vi "Motors.vi"() -> ()   [LabVIEW 2018]
doc: "The myRIO Project template acquires acceleration data from the onboard accelerometer and displays the changes of acceleration values in a waveform chart."
uses:
  <vilib>/Studica/Studica Toolkit/Background/Mxp Selection.ctl
  <vilib>/robotics/Steering/Wheel/Rotation Direction.ctl
  <vilib>/robotics/Steering/Wheel/Wheel Parameters.ctl
  <vilib>/robotics/Steering/Omnidirectional Wheel/NI_Robotics_Omnidirectional Wheel.lvclass
  C:/Program Files (x86)/National Instruments/LabVIEW 2018/vi.lib/robotics/Steering/Wheel/NI_Robotics_Wheel.lvclass
  <vilib>/robotics/Steering/Omnidirectional Wheel/Create Omnidirectional Wheel.vi
  <vilib>/robotics/Steering/Steering Frame/Create User Defined Steering Frame.vi
  <vilib>/addons/control/pid/pid.llb/PID (DBL).vi
  <vilib>/robotics/Steering/Steering Frame/NI_Robotics_Steering Frame.lvclass
  <vilib>/robotics/Steering/Wheel/NI_Robotics_Wheel.lvclass
  <vilib>/addons/control/pid/NI_PID_pid.lvlib
panel:
  out "Etu":cluster{"initial PV":dbl, "SP:":dbl}(graph)={"initial PV"=0.0, "SP:"=-0.0}
  in  "PID gains":T1={"proportional gain (Kc)"=1.0, "integral time (Ti, min)"=0.01, "derivative time (Td, min)"=0.0} {"derivative time (Td, min)" format="%.3f"; "integral time (Ti, min)" format="%.3f"; "proportional gain (Kc)" format="%.3f"}
  in  "Reset Encoders":bool
  out "Radians/s":dbl[](array[numeric])
  out "Up":bool
  out "Down":bool
  out "Speed":dbl
  out "Q":bool
  out "E":bool
  out "D":bool
  out "S":bool
  out "A":bool
  out "W":bool
  out "Keys":i16[](array[numeric])
  in  "Control Type":string(combo)="Keyboard"
  in  "Stop Button":bool
  in  "Angular Velocity (rad/s)":dbl(slide) min=-1.0 max=1.0 scale=1.0..-1.0
  out "Angular Velocity Feedback":dbl(slide) scale=1.0..-1.0
  in  "Y Velocity (m/s)":dbl(slide) min=-1.0 max=1.0 scale=-1.0..1.0
  out "Y Velocity Feedback":dbl(slide) scale=-1.0..1.0
  in  "X Velocity (m/s)":dbl(slide) min=-1.0 max=1.0 scale=-1.0..1.0
  out "X Velocity Feedback":dbl(slide) scale=-1.0..1.0
  in  "Not-Connected":dbl(slide) scale=-1.0..1.0
  in  "Oikea":dbl(slide)=-0.0 scale=-1.0..1.0
  in  "Vasen":dbl(slide)=-0.0 scale=-1.0..1.0
  in  "Etu":dbl(slide)=-0.0 scale=-1.0..1.0
  # "Keyboard"
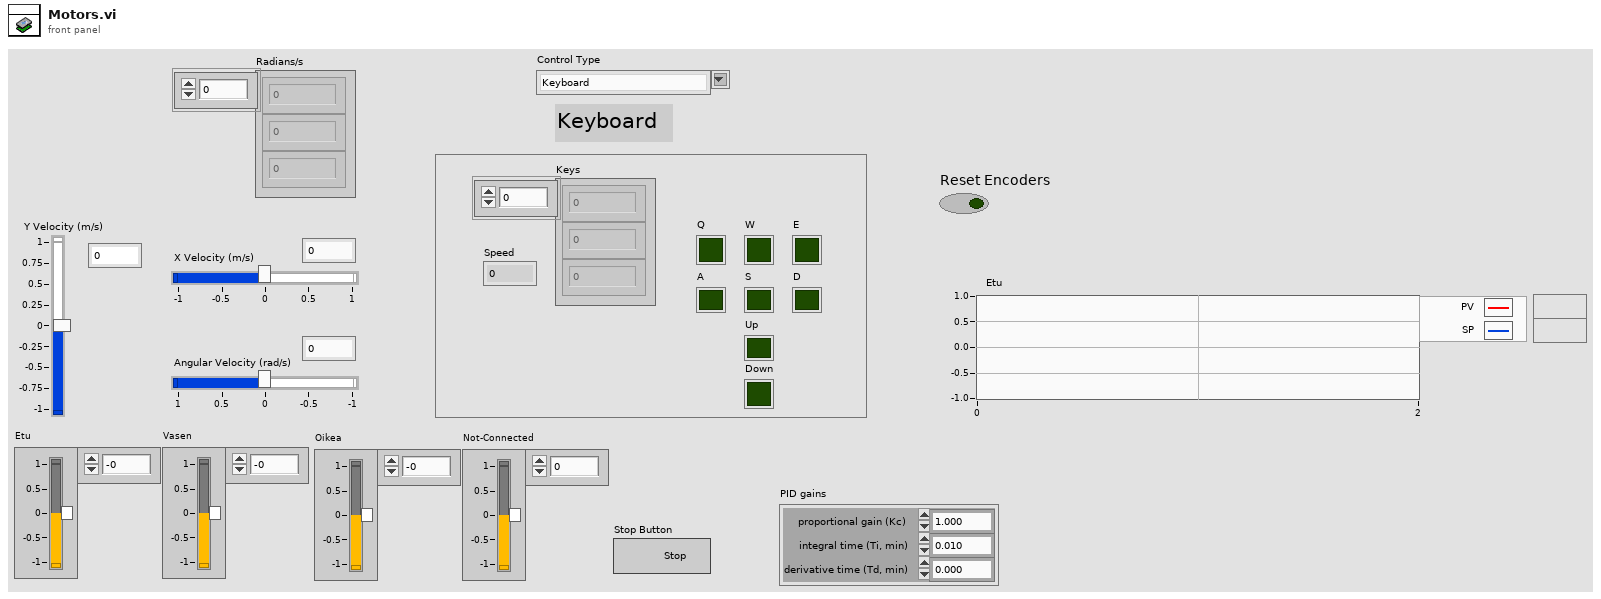
[diagram p1: front panel]
types:
  T1 = cluster{"proportional gain (Kc)":dbl, "integral time (Ti, min)":dbl, "derivative time (Td, min)":dbl}
  T2 = typedef "Mxp Selection.ctl" = enum16{"MXP A", "MXP B"}
  T3 = cluster{bool, "Tick Count(uSec)":u32, "Counter Value":i32[], "x-y":i32[]}
  T4 = typedef "NI_Robotics_Wheel.lvclass/Wheel Parameters.ctl" = cluster{"wheel radius":dbl, "gear ratio":dbl, "forward rotation direction":T5}
  T5 = typedef "NI_Robotics_Wheel.lvclass/Rotation Direction.ctl" = u16
  T6 = cluster{"Position":i32[], "Velocity RPM":dbl[], "Velocity RPS":dbl[], "Radians/s":dbl[]}
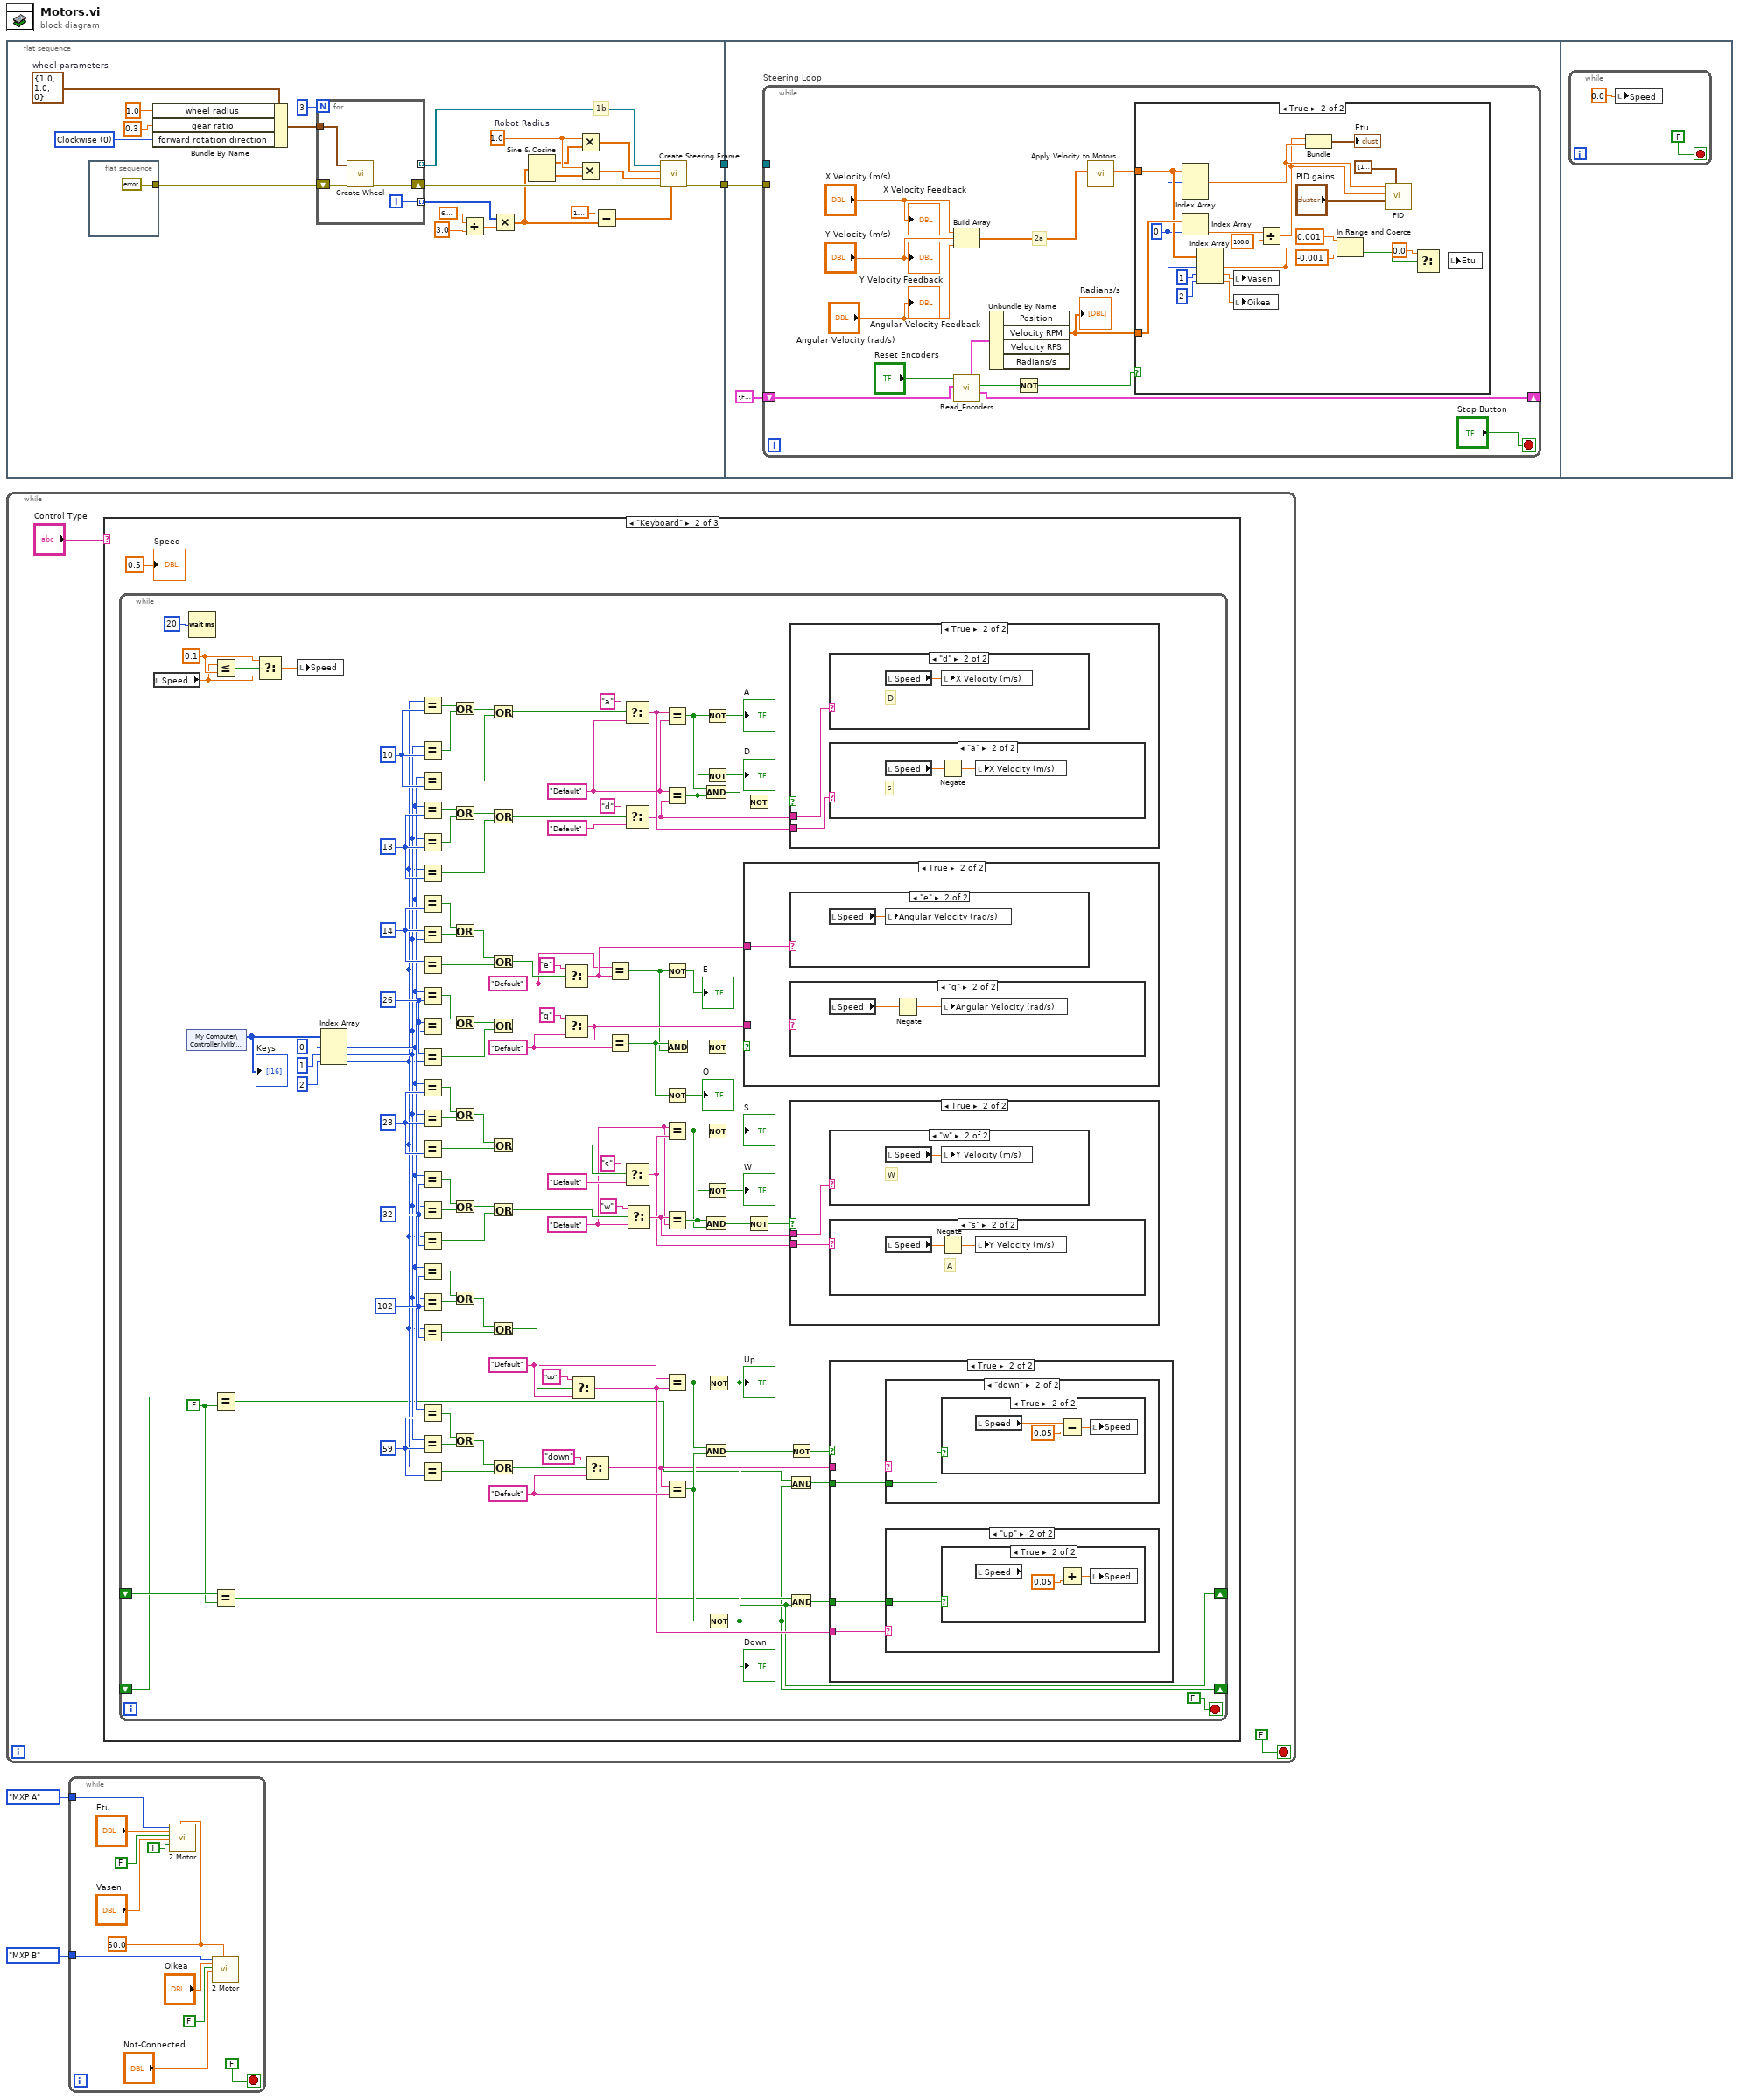
[diagram p0: block diagram]
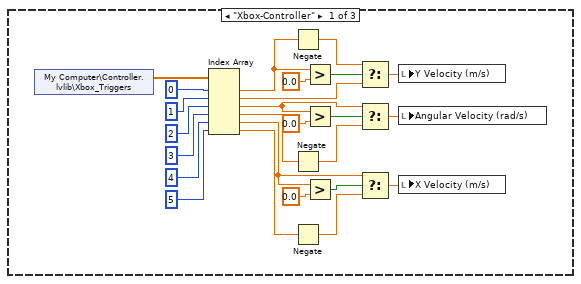
[diagram p3: hidden frame]
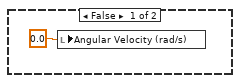
[diagram p9: hidden frame]
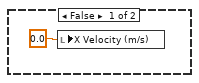
[diagram p12: hidden frame]
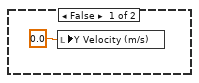
[diagram p15: hidden frame]
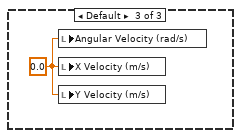
[diagram p18: hidden frame]
diagram:
  n1 = flat-sequence {
    tunnel: [w27] -> w2
    tunnel: [w8] -> w1
    tunnel: w2 -> [w34]
    tunnel: w1 -> [w36]
    frame #0 {
      w26 = T4 {"wheel radius"=1.0, "gear ratio"=1.0, "forward rotation direction"=0}  # wheel parameters
      w11 = T5 0 items=["Clockwise", "Counterclockwise"] ("forward rotation direction")
      w16 = 1.0  # Robot Radius
      # "1b"
      n2 = flat-sequence {
        tunnel: [errorcluster {"status"=FALSE, "code"=0, "source"=""} ("error out")] -> w22
        frame #0 {
        }
      }
      n3 = Bundle By Name(cluster=w26, "wheel radius"=1.0, "gear ratio"=0.3, "forward rotation direction"=w11) -> (w23:T4)
      n4 = for {
        N: 3 -> [_]
        shift-right: [w32] -> w9
        shift-left: w22 -> [w33]
        tunnel: [w31] -> w21 mode=indexing
        tunnel: w23 -> [w30]
        tunnel: [w29] -> w17 mode=indexing
        i -> [w29]
        n5 = call-poly <vilib>:"Create Wheel.vi"("error in (no error)"=w33, "wheel parameters"=w30) -> ("error out"=w32:errorcluster, "omni wheel out"=w31:refnum<class "NI_Robotics_Omnidirectional Wheel.lvclass">)  [unwired: 8 in]
      }
      n6 = Divide(x=6.283185307179586, y=3.0) -> (x/y=w18:dbl)
      n7 = Multiply(x=w17, y=w18) -> (x*y=w7:dbl[])
      n8 = Sine & Cosine(0:w7) -> (1:w6:dbl[], 2:w5:dbl[])
      n9 = Multiply(x=w16, y=w6) -> (x*y=w15:dbl[])
      n10 = Multiply(x=w16, y=w5) -> (x*y=w14:dbl[])
      n11 = Subtract(x=1.5707963267948966, y=w7) -> (x-y=w12:dbl[])
      n12 = call-poly <vilib>:"Create Steering Frame.vi"("wheel frame angles (rad)"=w12, "error in (no error)"=w9, "wheel y positions"=w14, "wheel x positions"=w15, "wheels"=w21) -> ("error out"=w8:errorcluster, "steering frame out"=w27:refnum<class "NI_Robotics_Steering Frame.lvclass">)  [unwired: 5 in]
    }
    frame #1 {
      n13 = while "Steering Loop" {
        tunnel: w36 -> [_]
        shift-right: [w42] -> _
        shift-left: T3 {FALSE, "Tick Count(uSec)"=0, "Counter Value"=[0, 0, 0, 0], "x-y"=[0, 0, 0, 0]} ("Cluster in") -> [w44]
        tunnel: w34 -> [w45]
        stop <- "Stop Button" stop-if-true
        # "2a"
        n14 = Build Array("X Velocity (m/s)", "Y Velocity (m/s)", "Angular Velocity (rad/s)") -> (w46:dbl[])
        n15 = call "Read_Encoders.vi"("Cluster in"=w44, "Reset Encoders"="Reset Encoders") -> ("Cluster Out"=w42:T3, "Updated"=w41:bool, "output cluster"=w43:T6)  [unwired: 5 in, 2 out]
        n16 = Unbundle By Name(w43) -> ("Velocity RPM"=w38:dbl[])  [unwired: 3 out]
        "Radians/s" <- w38
        n17 = Not(x=w41) -> (.not. x?=w40:bool)
        n18 = call-poly <vilib>:"Apply Velocity to Motors.vi"("steering frame velocity"=w46, "steering frame in"=w45) -> ("ccw motor velocity setpoints"=w39:dbl[])  [unwired: 5 in, 4 out]
        n19 = case shown="True" w40 {
          tunnel: w38 -> [_ w70]
          tunnel: w39 -> [_ w62]
          frame False {
          }
          frame True {
            w61 = 0 ("index")
            n20 = Index Array(array=w62, index #1=w61) -> (element #1=w67:dbl)  [unwired: 2 in, 2 out]
            n21 = Index Array(array=w70, index=w61) -> (element=w65:dbl)
            n22 = Index Array(array=w62, index #1=w61, index #2=1 ("index"), index #3=2 ("index")) -> (element #1=w51:dbl, element #2=w58:dbl, element #3=w57:dbl)
            n23 = local write "Vasen"(w58) -> ()
            n24 = local write "Oikea"(w57) -> ()
            n25 = Divide(x=w65, y=100.0) -> (x/y=w63:dbl)
            n26 = Bundle(w63, "Numeric"=w67) -> (→"Etu":cluster{dbl, "Numeric":dbl})  [unwired: 1 in]
            n27 = In Range and Coerce(upper limit=0.001, x=w51, lower limit=-0.001 ("upper limit")) -> (In Range?=w54:bool)  [unwired: 1 out]
            n28 = call-poly <vilib>:"PID.vi"("output range"=cluster{"output high":dbl, "output low":dbl} {"output high"=1.0, "output low"=-1.0}, "PID gains"="PID gains", "process variable"=w63, "setpoint"=w67) -> ()  [unwired: 6 in, 2 out]
            n29 = Select(t=0.0, s=w54, f=w51) -> (s? t:f=w52:dbl)
            n30 = local write "Etu"(w52) -> ()
          }
        }
        "X Velocity Feedback" <- "X Velocity (m/s)"
        "Y Velocity Feedback" <- "Y Velocity (m/s)"
        "Angular Velocity Feedback" <- "Angular Velocity (rad/s)"
      }
    }
    frame #2 {
      n31 = while {
        stop <- FALSE stop-if-true
        n32 = local write "Speed"(0.0 ("Speed")) -> ()
      }
    }
  }
  n33 = while {
    stop <- FALSE stop-if-true
    n34 = case shown="\"Keyboard\"" "Control Type" {
      frame "Xbox-Controller" {
        n35 = shared-variable "My Computer\\Controller.lvlib\\Xbox_Triggers"() -> (w99:dbl[])  [unwired: 1 in, 1 out]
        n36 = Index Array(array=w99, index #1=0 ("index"), index #2=1 ("index"), index #3=2 ("index"), index #4=3 ("index"), index #5=4 ("index"), index #6=5 ("index")) -> (element #1=w92:dbl, element #2=w91:dbl, element #3=w83:dbl, element #4=w81:dbl, element #5=w75:dbl, element #6=w76:dbl)
        n37 = Negate(x=w92) -> (-x=w93:dbl)
        n38 = Negate(x=w81) -> (-x=w82:dbl)
        n39 = Negate(x=w76) -> (-x=w77:dbl)
        n40 = Greater?(x=w92, y=0.0) -> (0:w95:bool)
        n41 = Greater?(x=w83, y=0.0) -> (0:w86:bool)
        n42 = Greater?(x=w75, y=0.0) -> (0:w80:bool)
        n43 = Select(t=w93, s=w95, f=w91) -> (s? t:f=w96:dbl)
        n44 = Select(t=w83, s=w86, f=w82) -> (s? t:f=w84:dbl)
        n45 = Select(t=w75, s=w80, f=w77) -> (s? t:f=w78:dbl)
        n46 = local write "Y Velocity (m/s)"(w96) -> ()
        n47 = local write "Angular Velocity (rad/s)"(w84) -> ()
        n48 = local write "X Velocity (m/s)"(w78) -> ()
      }
      frame "Keyboard" {
        n49 = while {
          shift-right: [w109] -> _
          shift-left: _ -> [w110]
          shift-right: [w102] -> _
          shift-left: _ -> [w107]
          stop <- FALSE stop-if-true
          w106 = FALSE ("y")
          w118 = "Default"
          w117 = "Default"
          w134 = 102 ("index")
          w135 = 59 ("index")
          w138 = 0.1 ("y")
          w155 = "Default"
          w165 = 14 ("index")
          w154 = "Default"
          w172 = 26 ("index")
          w185 = 13 ("index")
          w186 = 10 ("index")
          w174 = "Default"
          w199 = 28 ("index")
          w207 = 32 ("index")
          w182 = "Default"
          n50 = local read "Speed"() -> (w137:dbl)
          n51 = shared-variable "My Computer\\Controller.lvlib\\Keys"() -> (w213:i16[])  [unwired: 1 in, 1 out]
          "Keys" <- w213
          n52 = Wait (ms)(milliseconds to wait=u32 20) -> ()  [unwired: 1 out]
          n53 = Less Or Equal?(x=w137, y=w138) -> (x <= y?=w139:bool)
          n54 = Equal?(x=w107, y=w106) -> (x = y?=w103:bool)
          n55 = Equal?(x=w110, y=w106) -> (x = y?=w105:bool)
          n56 = Select(t=w138, s=w139, f=w137) -> (s? t:f=w136:dbl)
          n57 = local write "Speed"(w136) -> ()
          n58 = Index Array(array=w213, index #1=0 ("index"), index #2=1 ("index"), index #3=2 ("index")) -> (element #1=w133:i16, element #2=w132:i16, element #3=w131:i16)
          n59 = Equal?(x=w131, y=w186) -> (x = y?=w198:bool)
          n60 = Equal?(x=w132, y=w186) -> (x = y?=w197:bool)
          n61 = Equal?(x=w133, y=w186) -> (x = y?=w196:bool)
          n62 = Equal?(x=w133, y=w185) -> (x = y?=w192:bool)
          n63 = Equal?(x=w132, y=w185) -> (x = y?=w191:bool)
          n64 = Equal?(x=w131, y=w185) -> (x = y?=w190:bool)
          n65 = Equal?(x=w133, y=w165) -> (x = y?=w164:bool)
          n66 = Equal?(x=w165, y=w132) -> (x = y?=w163:bool)
          n67 = Equal?(x=w165, y=w131) -> (x = y?=w162:bool)
          n68 = Equal?(x=w133, y=w172) -> (x = y?=w171:bool)
          n69 = Equal?(x=w172, y=w132) -> (x = y?=w170:bool)
          n70 = Equal?(x=w172, y=w131) -> (x = y?=w169:bool)
          n71 = Equal?(x=w133, y=w199) -> (x = y?=w206:bool)
          n72 = Equal?(x=w132, y=w199) -> (x = y?=w205:bool)
          n73 = Equal?(x=w131, y=w199) -> (x = y?=w204:bool)
          n74 = Equal?(x=w133, y=w207) -> (x = y?=w212:bool)
          n75 = Equal?(x=w132, y=w207) -> (x = y?=w211:bool)
          n76 = Equal?(x=w131, y=w207) -> (x = y?=w210:bool)
          n77 = Equal?(x=w133, y=w134) -> (x = y?=w126:bool)
          n78 = Equal?(x=w132, y=w134) -> (x = y?=w127:bool)
          n79 = Equal?(x=w131, y=w134) -> (x = y?=w128:bool)
          n80 = Equal?(x=w133, y=w135) -> (x = y?=w125:bool)
          n81 = Equal?(x=w132, y=w135) -> (x = y?=w124:bool)
          n82 = Equal?(x=w131, y=w135) -> (x = y?=w123:bool)
          n83 = Or(x=w198, y=w197) -> (x .or. y?=w195:bool)
          n84 = Or(x=w192, y=w191) -> (x .or. y?=w189:bool)
          n85 = Or(x=w164, y=w163) -> (x .or. y?=w166:bool)
          n86 = Or(x=w171, y=w170) -> (x .or. y?=w173:bool)
          n87 = Or(x=w206, y=w205) -> (x .or. y?=w203:bool)
          n88 = Or(x=w212, y=w211) -> (x .or. y?=w209:bool)
          n89 = Or(x=w126, y=w127) -> (x .or. y?=w129:bool)
          n90 = Or(x=w125, y=w124) -> (x .or. y?=w130:bool)
          n91 = Or(x=w195, y=w196) -> (x .or. y?=w194:bool)
          n92 = Or(x=w189, y=w190) -> (x .or. y?=w188:bool)
          n93 = Or(x=w166, y=w162) -> (x .or. y?=w160:bool)
          n94 = Or(x=w173, y=w169) -> (x .or. y?=w167:bool)
          n95 = Or(x=w203, y=w204) -> (x .or. y?=w202:bool)
          n96 = Or(x=w209, y=w210) -> (x .or. y?=w208:bool)
          n97 = Or(x=w129, y=w128) -> (x .or. y?=w120:bool)
          n98 = Or(x=w130, y=w123) -> (x .or. y?=w119:bool)
          n99 = Select(t="e", s=w160, f=w155) -> (s? t:f=w156:string)
          n100 = Select(t="q", s=w167, f=w154) -> (s? t:f=w157:string)
          n101 = Select(t="up", s=w120, f=w118) -> (s? t:f=w112:string)
          n102 = Select(t="down", s=w119, f=w117) -> (s? t:f=w111:string)
          n103 = Equal?(x=w155, y=w156) -> (x = y?=w140:bool)
          n104 = Equal?(x=w157, y=w154) -> (x = y?=w143:bool)
          n105 = Select(t="a", s=w194, f=w174) -> (s? t:f=w176:string)
          n106 = Select(t="d", s=w188, f="Default") -> (s? t:f=w175:string)
          n107 = Select(t="s", s=w202, f="Default") -> (s? t:f=w183:string)
          n108 = Select(t="w", s=w208, f=w182) -> (s? t:f=w184:string)
          n109 = Equal?(x=w176, y=w174) -> (x = y?=w146:bool)
          n110 = Equal?(x=w174, y=w175) -> (x = y?=w144:bool)
          n111 = Not(x=w140) -> (.not. x?=→"E":bool)
          n112 = Not(x=w143) -> (.not. x?=→"Q":bool)
          n113 = Equal?(x=w182, y=w183) -> (x = y?=w148:bool)
          n114 = Equal?(x=w184, y=w182) -> (x = y?=w151:bool)
          n115 = Equal?(x=w118, y=w112) -> (x = y?=w115:bool)
          n116 = Equal?(x=w111, y=w117) -> (x = y?=w114:bool)
          n117 = And(x=w143, y=w140) -> (x .and. y?=w159:bool)
          n118 = And(x=w146, y=w144) -> (x .and. y?=w178:bool)
          n119 = And(x=w151, y=w148) -> (x .and. y?=w181:bool)
          n120 = And(x=w115, y=w114) -> (x .and. y?=w116:bool)
          n121 = Not(x=w146) -> (.not. x?=→"A":bool)
          n122 = Not(x=w144) -> (.not. x?=→"D":bool)
          n123 = Not(x=w159) -> (.not. x?=w158:bool)
          n124 = Not(x=w148) -> (.not. x?=→"S":bool)
          n125 = Not(x=w151) -> (.not. x?=→"W":bool)
          n126 = Not(x=w115) -> (.not. x?=w109:bool)
          "Up" <- w109
          n127 = Not(x=w114) -> (.not. x?=w102:bool)
          "Down" <- w102
          n128 = case shown="True" w158 {
            tunnel: w156 -> [_ w231]
            tunnel: w157 -> [_ w230]
            frame False {
              n129 = local write "Angular Velocity (rad/s)"(0.0 ("t")) -> ()
            }
            frame True {
              n130 = case shown="\"e\"" w231 {
                frame "False", Default {
                }
                frame "e" {
                  n131 = local read "Speed"() -> (w232:dbl)
                  n132 = local write "Angular Velocity (rad/s)"(w232) -> ()
                }
              }
              n133 = case shown="\"q\"" w230 {
                frame "False", Default {
                }
                frame "q" {
                  n134 = local read "Speed"() -> (w234:dbl)
                  n135 = Negate(x=w234) -> (-x=w233:dbl)
                  n136 = local write "Angular Velocity (rad/s)"(w233) -> ()
                }
              }
            }
          }
          n137 = Not(x=w178) -> (.not. x?=w177:bool)
          n138 = Not(x=w181) -> (.not. x?=w180:bool)
          n139 = Not(x=w116) -> (.not. x?=w113:bool)
          n140 = And(x=w103, y=w102) -> (x .and. y?=w104:bool)
          n141 = And(x=w105, y=w109) -> (x .and. y?=w108:bool)
          n142 = case shown="True" w177 {
            tunnel: w176 -> [_ w237]
            tunnel: w175 -> [_ w236]
            frame False {
              n143 = local write "X Velocity (m/s)"(0.0 ("t")) -> ()
            }
            frame True {
              n144 = case shown="\"d\"" w236 {
                frame "False", Default {
                }
                frame "d" {
                  # "D"
                  n145 = local read "Speed"() -> (w238:dbl)
                  n146 = local write "X Velocity (m/s)"(w238) -> ()
                }
              }
              n147 = case shown="\"a\"" w237 {
                frame "False", Default {
                }
                frame "a" {
                  # "S"
                  n148 = local read "Speed"() -> (w240:dbl)
                  n149 = Negate(x=w240) -> (-x=w239:dbl)
                  n150 = local write "X Velocity (m/s)"(w239) -> ()
                }
              }
            }
          }
          n151 = case shown="True" w180 {
            tunnel: w184 -> [_ w243]
            tunnel: w183 -> [_ w242]
            frame False {
              n152 = local write "Y Velocity (m/s)"(0.0 ("t")) -> ()
            }
            frame True {
              n153 = case shown="\"w\"" w243 {
                frame "False", Default {
                }
                frame "w" {
                  # "W"
                  n154 = local read "Speed"() -> (w246:dbl)
                  n155 = local write "Y Velocity (m/s)"(w246) -> ()
                }
              }
              n156 = case shown="\"s\"" w242 {
                frame "False", Default {
                }
                frame "s" {
                  # "A"
                  n157 = local read "Speed"() -> (w244:dbl)
                  n158 = Negate(x=w244) -> (-x=w245:dbl)
                  n159 = local write "Y Velocity (m/s)"(w245) -> ()
                }
              }
            }
          }
          n160 = case shown="True" w113 {
            tunnel: w112 -> [_ w220]
            tunnel: w111 -> [_ w219]
            tunnel: w108 -> [_ w218]
            tunnel: w104 -> [_ w217]
            frame False {
            }
            frame True {
              n161 = case shown="\"down\"" w219 {
                tunnel: w217 -> [_ w221]
                frame "False", Default {
                }
                frame "down" {
                  n162 = case shown="True" w221 {
                    frame False {
                    }
                    frame True {
                      n163 = local read "Speed"() -> (w223:dbl)
                      n164 = Subtract(x=w223, y=0.05) -> (x-y=w222:dbl)
                      n165 = local write "Speed"(w222) -> ()
                    }
                  }
                }
              }
              n166 = case shown="\"up\"" w220 {
                tunnel: w218 -> [_ w225]
                frame "False", Default {
                }
                frame "up" {
                  n167 = case shown="True" w225 {
                    frame False {
                    }
                    frame True {
                      n168 = local read "Speed"() -> (w228:dbl)
                      n169 = Add(x=w228, y=0.05) -> (x+y=w226:dbl)
                      n170 = local write "Speed"(w226) -> ()
                    }
                  }
                }
              }
            }
          }
        }
        "Speed" <- 0.5 ("Speed")
      }
      frame Default {
        w247 = 0.0 ("Angular Velocity (rad/s)")
        n171 = local write "Angular Velocity (rad/s)"(w247) -> ()
        n172 = local write "X Velocity (m/s)"(w247) -> ()
        n173 = local write "Y Velocity (m/s)"(w247) -> ()
      }
    }
  }
  n174 = while {
    tunnel: Mxp_Selection."MXP A" ("Mxp Side") -> [w258]
    tunnel: Mxp_Selection."MXP B" ("Mxp Side") -> [w257]
    stop <- FALSE stop-if-true
    w252 = 50.0 ("Frequency [Hz]")
    n175 = call <vilib>:"2 Motor.vi"("Mxp Side"=w258, "Speed M0"="Etu", "Invert M0"=FALSE, "Speed M1"="Vasen", "Invert M1"=TRUE ("Invert M0"), "Frequency [Hz]"=w252) -> ()  [unwired: 13 in, 1 out]
    n176 = call <vilib>:"2 Motor.vi"("Mxp Side"=w257, "Speed M0"="Oikea", "Invert M0"=FALSE, "Speed M1"="Not-Connected", "Frequency [Hz]"=w252) -> ()  [unwired: 14 in, 1 out]
  }
